vi "test-find-path-debug.vi"() -> ()   [LabVIEW 2019]
uses:
  <vilib>/Rock Robotics/WPI/ThirdParty/JAS_Junk/TrajLib/TypeDef/TRANSLATION2D.ctl
  <vilib>/Rock Robotics/WPI/ThirdParty/MJansen/PathPlanner/TypeDef/PathPlannerGoalEndState.ctl
  <vilib>/Rock Robotics/WPI/ThirdParty/JAS_Junk/TrajLib/TypeDef/ROTATION2D.ctl
  <vilib>/Rock Robotics/WPI/ThirdParty/MJansen/PathPlanner/TypeDef/PathPlannerPath.ctl
  <vilib>/Rock Robotics/WPI/ThirdParty/MJansen/PathPlanner/TypeDef/PathPlannerRotationTarget.ctl
  <vilib>/Rock Robotics/WPI/ThirdParty/MJansen/PathPlanner/TypeDef/PathPlannerConstraintsZone.ctl
  <vilib>/Rock Robotics/WPI/ThirdParty/MJansen/PathPlanner/TypeDef/PathPlannerPathConstraints.ctl
  <vilib>/Rock Robotics/WPI/ThirdParty/MJansen/PathPlanner/TypeDef/PathPlannerEventMarker.ctl
  <vilib>/Rock Robotics/WPI/ThirdParty/MJansen/PathPlanner/TypeDef/PathPlannerCommandUtil.ctl
  <vilib>/Rock Robotics/WPI/ThirdParty/MJansen/PathPlanner/ENum/PathPlanner_CommandUtilType_ENUM.ctl
  <vilib>/Rock Robotics/WPI/ThirdParty/MJansen/PathPlanner/TypeDef/PathPlannerPathPoint.ctl
  <vilib>/Rock Robotics/WPI/ThirdParty/MJansen/PathPlanner/TypeDef/PathPlannerWaypoint.ctl
  <vilib>/Rock Robotics/WPI/ThirdParty/MJansen/PathPlanner/TypeDef/PathPlannerPointTowardsZone.ctl
  <vilib>/Rock Robotics/WPI/ThirdParty/MJansen/PathPlanner/TypeDef/PathPlannerIdealStartingState.ctl
  <vilib>/Rock Robotics/WPI/ThirdParty/JAS_Junk/TrajLib/TypeDef/CHASSIS_SPEEDS.ctl
  <vilib>/Rock Robotics/WPI/ThirdParty/MJansen/PathPlanner/VI/PathPlanner_GridPosition_Get.vi
  <vilib>/Rock Robotics/WPI/ThirdParty/JAS_Junk/TrajLib/Translation2d_Create.vi
  <vilib>/Rock Robotics/WPI/ThirdParty/MJansen/PathPlanner/VI/PathPlanner_PathFinder_Globals.vi
  <vilib>/robotics/Navigation/shared/WorldMap/OccupancyGridWorldMap/NI_Robotics_OccupancyGridWorldMap.lvclass
  <vilib>/robotics/Navigation/shared/MapNode/AbstractDstarNode/NI_Robotics_AbstractDstarNode.lvclass
  <vilib>/Rock Robotics/WPI/ThirdParty/MJansen/PathPlanner/PathPlanner24.lvlib
  <vilib>/Rock Robotics/WPI/ThirdParty/JAS_Junk/TrajLib/Trajectory_Library.lvlib
panel:
  out "Loop Count 2":i32
  out "Extract Simplified Path Size":i32
  out "Do Reset Err Count":i64
  out "Do Minor Err Count":i64
  out "Do Major Err Count":i64
  out "Extract Path Size":i32
  out "Field":cluster{dbl[], dbl[]}[](graph)
  out "Error_No_Path":bool
  out "New Path Available":bool
  out "Loop Count":i32
  out "TerminateWorker":bool
  out "Do Work Count":i64
  out "Do Reset Count":i64
  out "Do Minor Count":i64
  out "Do Major Count":i64
  out "PathPlannerPath":T1={"Reversed"=FALSE, "RotationTargets"=[], "ConstraintZones"=[], "EventMarkers"=[], "GlobalConstraints"={"MaxVelocityMps;"=0.0, "MaxAccelerationMpsSq;"=0.0, "MaxAngularVelRadPsEc;"=0.0, "MaxAngularAccRadPSecSq"=0.0, "Exists"=FALSE, "Unlimited"=FALSE, "NominalVoltageVolts"=1.0}, "GoalEndState"={"VelocityMPS"=0.0, "Rotation"={"VALUE"=0.0, "COS"=1.0, "SIN"=0.0}}, "AllPoints"=[], "Name"="", "Waypoints"=[], "PointTowardsZones"=[], "IdealStartingState"={"VelocityMPS"=0.0, "Rotation"={"VALUE"=0.0, "COS"=1.0, "SIN"=0.0}}, "IsChoreoPath"=FALSE, "PreventFlipping"=FALSE} {"IdealStartingState"."Rotation"."SIN" format="%13.4f"; "IdealStartingState"."Rotation"."COS" format="%13.4f"; "IdealStartingState"."Rotation"."VALUE" format="%13.4f"; "PointTowardsZones"."TargetPosition"."Y" format="%14.3f"; "PointTowardsZones"."TargetPosition"."X" format="%14.3f"; "PointTowardsZones"."RotationOffset"."SIN" format="%13.4f"; "PointTowardsZones"."RotationOffset"."COS" format="%13.4f"; "PointTowardsZones"."RotationOffset"."VALUE" format="%13.4f"; "Waypoints"."nextControl"."Y" format="%14.3f"; "Waypoints"."nextControl"."X" format="%14.3f"; "Waypoints"."anchor"."Y" format="%14.3f"; "Waypoints"."anchor"."X" format="%14.3f"; "Waypoints"."prevControl"."Y" format="%14.3f"; "Waypoints"."prevControl"."X" format="%14.3f"; "AllPoints"."RotationTarget"."rotation"."SIN" format="%13.4f"; "AllPoints"."RotationTarget"."rotation"."COS" format="%13.4f"; "AllPoints"."RotationTarget"."rotation"."VALUE" format="%13.4f"; "AllPoints"."Position"."Y" format="%14.3f"; "AllPoints"."Position"."X" format="%14.3f"; "GoalEndState"."Rotation"."SIN" format="%13.4f"; "GoalEndState"."Rotation"."COS" format="%13.4f"; "GoalEndState"."Rotation"."VALUE" format="%13.4f"; "RotationTargets"."rotation"."SIN" format="%13.4f"; "RotationTargets"."rotation"."COS" format="%13.4f"; "RotationTargets"."rotation"."VALUE" format="%13.4f"}
  in  "GoalEndState":T9={"VelocityMPS"=0.0, "Rotation"={"VALUE"=0.0, "COS"=1.0, "SIN"=0.0}} {"Rotation"."SIN" format="%13.4f"; "Rotation"."COS" format="%13.4f"; "Rotation"."VALUE" format="%13.4f"}
  in  "Goal Position":T11={"X"=14.0, "Y"=7.0} {"Y" step=0.25 format="%14.3f"; "X" step=0.25 format="%14.3f"}
  in  "StartPosition":T11={"X"=1.5, "Y"=1.5} {"Y" step=0.25 format="%14.3f"; "X" step=0.25 format="%14.3f"}
  out "NewPathAvailLastCheck":i32
  out "NewPathAvailCount":i32
  out "BackGroundInitialized":bool
  out "Main Program Name":string
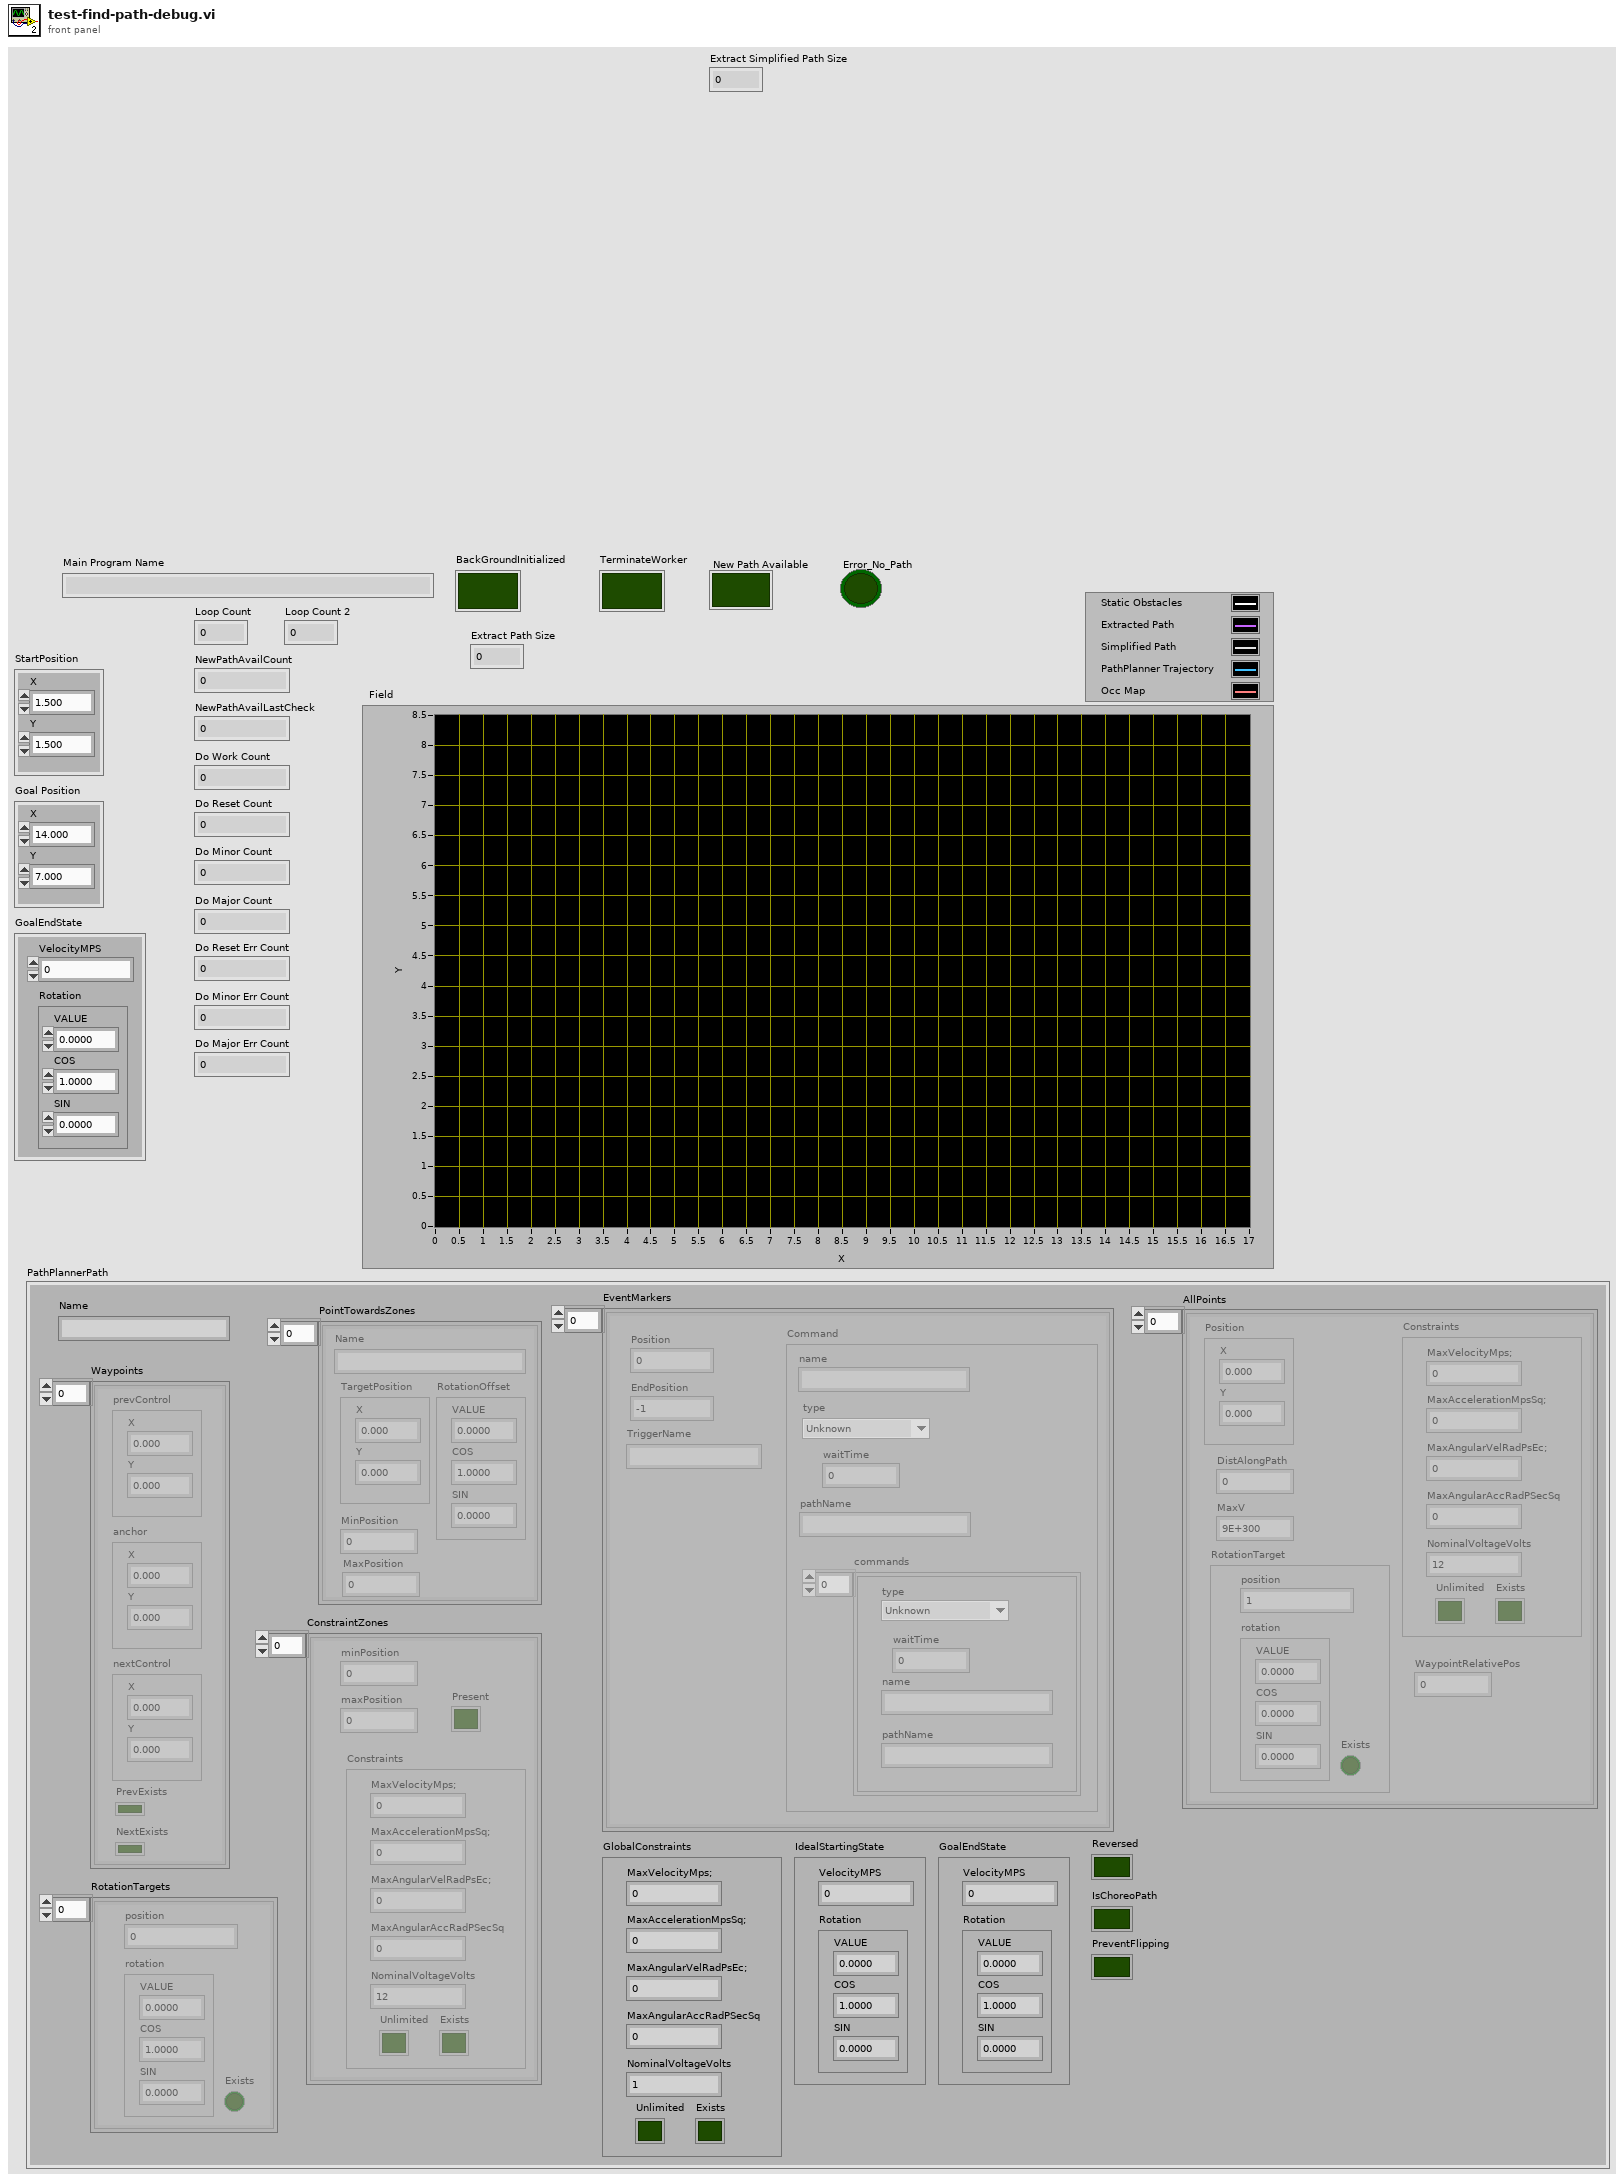
[diagram p1: front panel]
types:
  T1 = typedef "PathPlanner24.lvlib/PathPlannerPath.ctl" = cluster{"Reversed":bool, "RotationTargets":T2[], "ConstraintZones":T4[], "EventMarkers":T6[], "GlobalConstraints":T5, "GoalEndState":T9, "AllPoints":T10[], "Name":string, "Waypoints":T12[], "PointTowardsZones":T13[], "IdealStartingState":T14, "IsChoreoPath":bool, "PreventFlipping":bool}
  T2 = typedef "PathPlanner24.lvlib/PathPlannerRotationTarget.ctl" = cluster{"position":dbl, "rotation":T3, "Exists":bool}
  T3 = typedef "Trajectory_Library.lvlib/ROTATION2D.ctl" = cluster{"VALUE":dbl, "COS":dbl, "SIN":dbl}
  T4 = typedef "PathPlanner24.lvlib/PathPlannerConstraintsZone.ctl" = cluster{"minPosition":dbl, "maxPosition":dbl, "Constraints":T5, "Present":bool}
  T5 = typedef "PathPlanner24.lvlib/PathPlannerPathConstraints.ctl" = cluster{"MaxVelocityMps;":dbl, "MaxAccelerationMpsSq;":dbl, "MaxAngularVelRadPsEc;":dbl, "MaxAngularAccRadPSecSq":dbl, "Exists":bool, "Unlimited":bool, "NominalVoltageVolts":dbl}
  T6 = typedef "PathPlanner24.lvlib/PathPlannerEventMarker.ctl" = cluster{"Position":dbl, "Command":T7, "TriggerName":string, "EndPosition":dbl}
  T7 = typedef "PathPlanner24.lvlib/PathPlannerCommandUtil.ctl" = cluster{"waitTime":dbl, "name":string, "pathName":string, "commands":cluster{"type":T8, "waitTime":dbl, "name":string, "pathName":string}[], "type":T8}
  T8 = typedef "PathPlanner24.lvlib/PathPlanner_CommandUtilType_ENUM.ctl" = enum16{"Unknown", "Wait", "Named", "Path", "Sequential", "Parallel", "Race", "Deadline"}
  T9 = typedef "PathPlanner24.lvlib/PathPlannerGoalEndState.ctl" = cluster{"VelocityMPS":dbl, "Rotation":T3}
  T10 = typedef "PathPlanner24.lvlib/PathPlannerPathPoint.ctl" = cluster{"Position":T11, "DistAlongPath":dbl, "MaxV":dbl, "Constraints":T5, "RotationTarget":T2, "WaypointRelativePos":dbl}
  T11 = typedef "Trajectory_Library.lvlib/TRANSLATION2D.ctl" = cluster{"X":dbl, "Y":dbl}
  T12 = typedef "PathPlanner24.lvlib/PathPlannerWaypoint.ctl" = cluster{"prevControl":T11, "anchor":T11, "nextControl":T11, "PrevExists":bool, "NextExists":bool}
  T13 = typedef "PathPlanner24.lvlib/PathPlannerPointTowardsZone.ctl" = cluster{"RotationOffset":T3, "Name":string, "TargetPosition":T11, "MinPosition":dbl, "MaxPosition":dbl}
  T14 = typedef "PathPlanner24.lvlib/PathPlannerIdealStartingState.ctl" = cluster{"VelocityMPS":dbl, "Rotation":T3}
  T15 = cluster{"DoResetErrCount":i64, "DoResetCount":i64, "DoMinorErrCount":i64, "DoMinorCount":i64, "DoMajorErrCount":i64, "DoMajorCount":i64, "DoWorkLoopCount":i64, "BackGroundInitialized":bool, "TerminateWorker":bool}
  T16 = typedef "Trajectory_Library.lvlib/CHASSIS_SPEEDS.ctl" = cluster{"vX":dbl, "vY":dbl, "vOmega":dbl}
  T17 = typedef "PathPlanner24.lvlib/PathPlannerFinderGridPosition.ctl" = cluster{"X":i32, "Y":i32}
  T18 = cluster{"ExtractedPath":T17[], "ExtractedPathSimplified":T17[], "ExtractedFieldPosPath":T11[], "CurrentPath":T11[], "Obstacles":set{T17}, "StaticOccupancyGrid":refnum<data-value>, "path references":refnum<data-value>[], "Main Program Name":string}
  T19 = typedef "PathPlanner24.lvlib/PathPlannerTrajectory.ctl" = cluster{"States":T20[]}
  T20 = typedef "PathPlanner24.lvlib/PathPlannerTrajectoryState.ctl" = cluster{"TimeSeconds":dbl, "VelocityMPS":dbl, "AccerationMpsSq":dbl, "HeadingAngularVelRadPerSec":dbl, "PositionMeters":T11, "Heading":T3, "TargetHolonomicRotation":T3, "CurvatureRadPerMeter":dbl, "PathPlannerConstraints":T5, "DeltaPos":dbl}
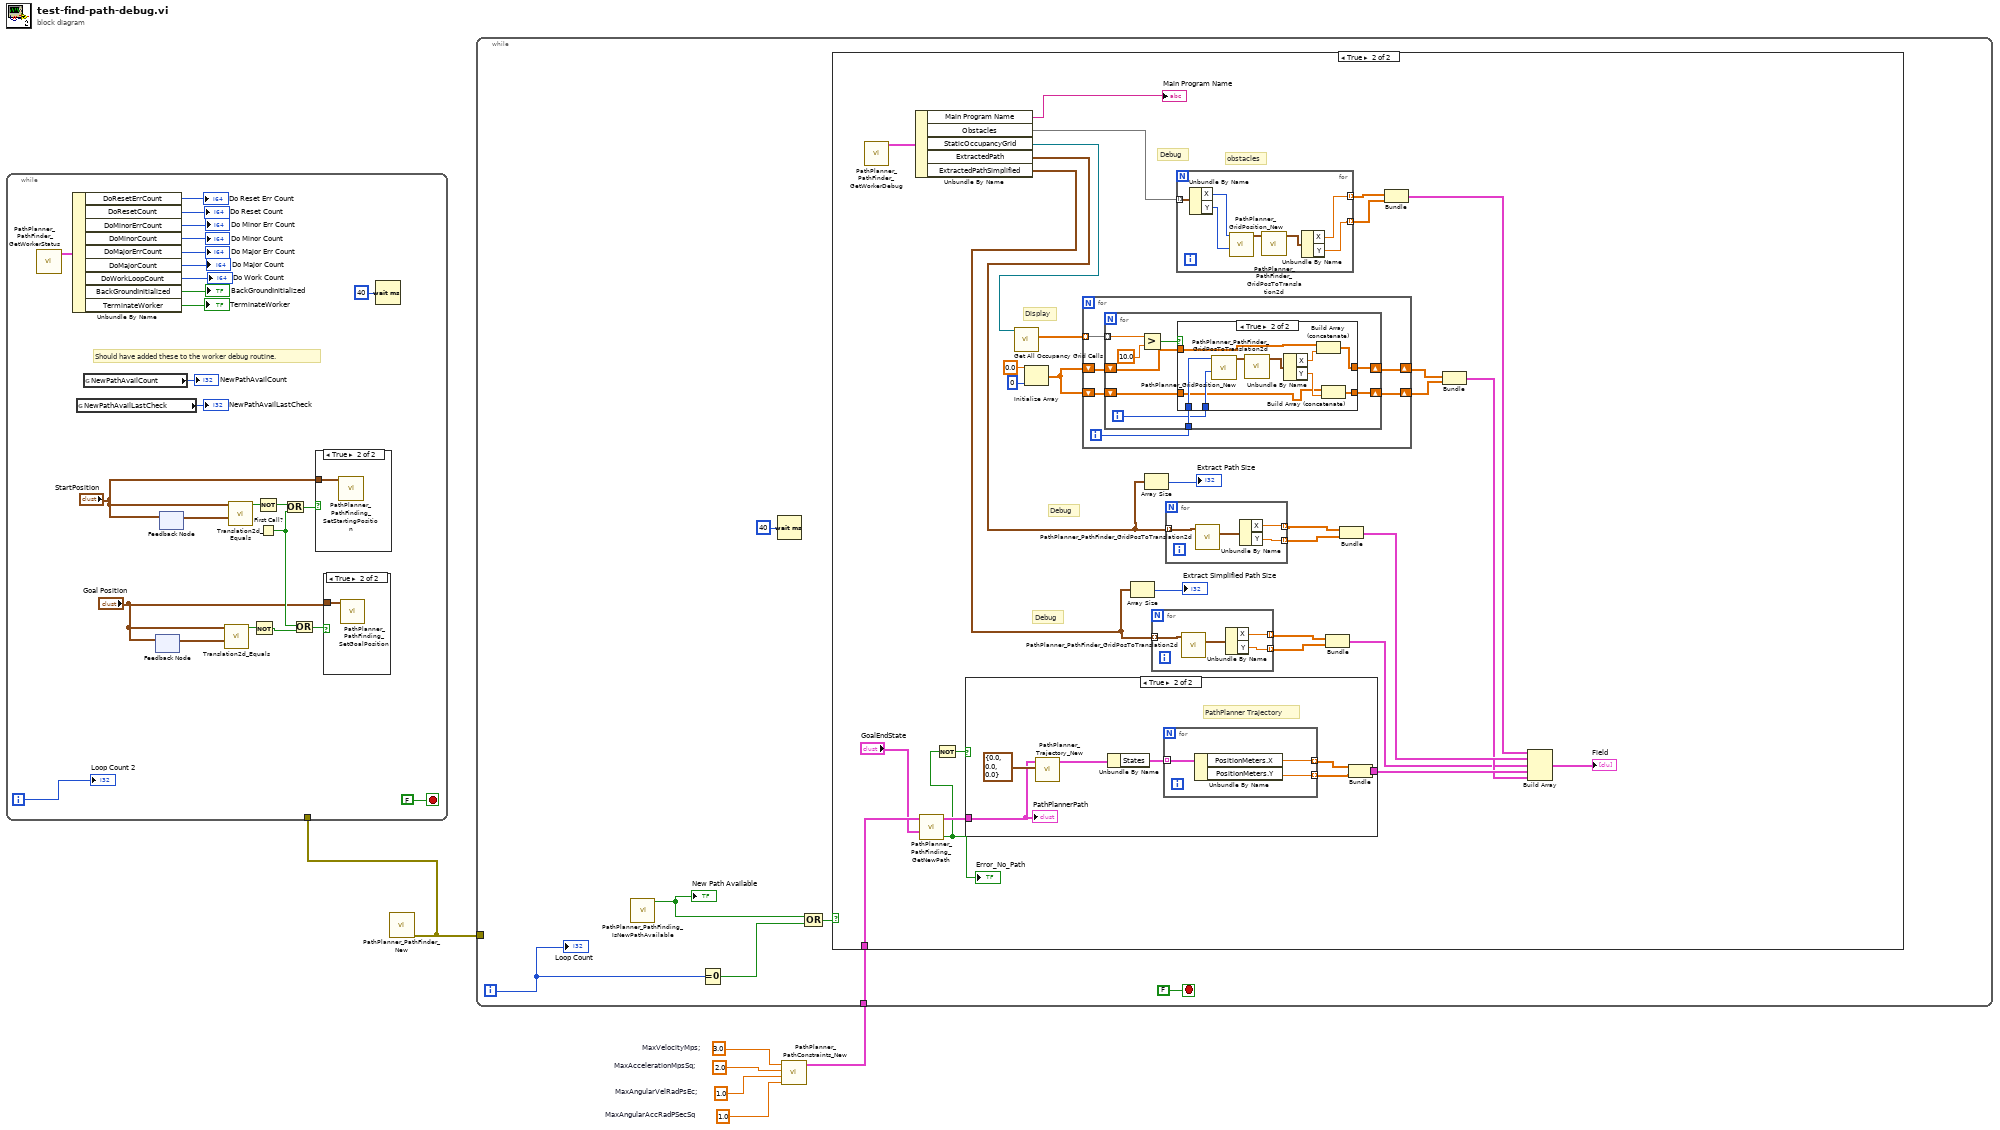
[diagram p0: block diagram]
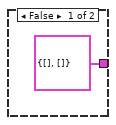
[diagram p5: hidden frame]
diagram:
  w2 = 3.0  # MaxVelocityMps;
  w3 = 2.0  # MaxAccelerationMpsSq;
  w4 = 1.0  # MaxAngularVelRadPsEc;
  w5 = 1.0  # MaxAngularAccRadPSecSq
  n1 = call <vilib>:"PathPlanner_PathFinder_New.vi"() -> ("error out"=w1:errorcluster)  [unwired: 11 in]
  n2 = while {
    tunnel: w1 -> [_]
    i -> [w18]
    stop <- FALSE stop-if-true
    # "Should have added these to the worker debug routine."
    n3 = call <vilib>:"PathPlanner_PathFinder_GetWorkerStatus.vi"() -> ("PathFindingWorkerStatus"=w23:T15)  [unwired: 11 in]
    n4 = Unbundle By Name(w23) -> ("DoResetErrCount"=→"Do Reset Err Count":i64, "DoResetCount"=→"Do Reset Count":i64, "DoMinorErrCount"=→"Do Minor Err Count":i64, "DoMinorCount"=→"Do Minor Count":i64, "DoMajorErrCount"=→"Do Major Err Count":i64, "DoMajorCount"=→"Do Major Count":i64, "DoWorkLoopCount"=→"Do Work Count":i64, "BackGroundInitialized"=→"BackGroundInitialized":bool, "TerminateWorker"=→"TerminateWorker":bool)
    n5 = global read "PathPlanner_PathFinder_Globals.vi" "NewPathAvailLastCheck"() -> (→"NewPathAvailLastCheck":i32)
    n6 = global read "PathPlanner_PathFinder_Globals.vi" "NewPathAvailCount"() -> (→"NewPathAvailCount":i32)
    n7 = feedback #1() -> (w9:T11)  [unwired: 1 in]
    n8 = feedback-in #1("Goal Position") -> ()
    n9 = feedback #2() -> (w7:T11)  [unwired: 1 in]
    n10 = feedback-in #2("StartPosition") -> ()
    n11 = call <vilib>:"Translation2d_Equals.vi"("other Translation"=w9, "In Translation"="Goal Position") -> ("Equals"=w10:bool)  [unwired: 9 in]
    n12 = call <vilib>:"Translation2d_Equals.vi"("other Translation"=w7, "In Translation"="StartPosition") -> ("Equals"=w8:bool)  [unwired: 9 in]
    n13 = Not(x=w10) -> (.not. x?=w15:bool)
    n14 = Not(x=w8) -> (.not. x?=w17:bool)
    n15 = First Call?() -> (First Call?: T/F=w16:bool)
    n16 = Or(x=w17, y=w16) -> (x .or. y?=w13:bool)
    n17 = Or(x=w16, y=w15) -> (x .or. y?=w14:bool)
    n18 = case shown="True" w13 {
      tunnel: "StartPosition" -> [_ w34]
      frame False {
      }
      frame True {
        n19 = call <vilib>:"PathPlanner_PathFinding_SetStartingPosition.vi"("StartPosition"=w34) -> ()  [unwired: 10 in, 1 out]
      }
    }
    n20 = case shown="True" w14 {
      tunnel: "Goal Position" -> [_ w33]
      frame False {
      }
      frame True {
        n21 = call <vilib>:"PathPlanner_PathFinding_SetGoalPosition.vi"("GoalPosition"=w33) -> ()  [unwired: 10 in, 1 out]
      }
    }
    n22 = Wait (ms)(milliseconds to wait=u32 40) -> ()  [unwired: 1 out]
    "Loop Count 2" <- w18
  }
  n23 = call <vilib>:"PathPlanner_PathConstraints_New.vi"("MaxAngularAccRadPSecSq"=w5, "MaxAngularVelRadPsEc;"=w4, "MaxAccelerationMpsSq;"=w3, "MaxVelocityMps;"=w2) -> ("PathPlannerConstraints"=w6:T5)  [unwired: 7 in]
  n24 = while {
    tunnel: w6 -> [w38]
    tunnel: w1 -> [_]
    i -> [w40]
    stop <- FALSE stop-if-true
    n25 = call <vilib>:"PathPlanner_PathFinding_IsNewPathAvailable.vi"() -> ("New Path Available"=w35:bool)  [unwired: 10 in, 1 out]
    "New Path Available" <- w35
    n26 = Equal To 0?(x=w40) -> (x = 0?=w37:bool)
    n27 = Wait (ms)(milliseconds to wait=u32 40) -> ()  [unwired: 1 out]
    n28 = Compound Arithmetic op=OR(w35, w37) -> (w39:bool)
    n29 = case shown="True" w39 {
      tunnel: w38 -> [_ w67]
      frame False {
      }
      frame True {
        # "Debug"
        # "Display"
        # "Debug"
        # "Debug"
        # "obstacles"
        n30 = call <vilib>:"PathPlanner_PathFinder_GetWorkerDebug.vi"() -> ("PathFinderWorkerDebug"=w49:T18)  [unwired: 11 in]
        n31 = Unbundle By Name(w49) -> ("Main Program Name"=→"Main Program Name":string, "Obstacles"=w47:set{T17}, "StaticOccupancyGrid"=w46:refnum<data-value>, "ExtractedPath"=w45:T17[], "ExtractedPathSimplified"=w44:T17[])
        n32 = call <vilib>:"PathPlanner_PathFinding_GetNewPath.vi"("GoalEndState"="GoalEndState", "PathPlannerPathConstraints"=w67) -> ("Error_No_Path"=w42:bool, "PathPlannerPath"=w65:T1)  [unwired: 8 in]
        "Error_No_Path" <- w42
        n33 = Not(x=w42) -> (.not. x?=w43:bool)
        n34 = case shown="True" w43 {
          tunnel: w65 -> [_ w78]
          tunnel: [cluster{dbl[], dbl[]} {[], []} w74] -> w62
          frame False {
          }
          frame True {
            # "PathPlanner Trajectory"
            n35 = call <vilib>:"PathPlanner_Trajectory_New.vi"("StartingSpeeds"=T16 {"vX"=0.0, "vY"=0.0, "vOmega"=0.0}, "Path"=w78) -> ("PathPlannerTrajectory"=w79:T19)  [unwired: 8 in, 1 out]
            n36 = Unbundle By Name(w79) -> ("States"=w77:T20[])
            n37 = for {
              tunnel: [w82] -> w76 mode=indexing
              tunnel: [w83] -> w75 mode=indexing
              tunnel: w77 -> [w81] mode=indexing
              n38 = Unbundle By Name(w81) -> ("PositionMeters.X"=w82:dbl, "PositionMeters.Y"=w83:dbl)
            }
            n39 = Bundle(w76, w75) -> (w74:cluster{dbl[], dbl[]})  [unwired: 1 in]
            "PathPlannerPath" <- w78
          }
        }
        n40 = call <vilib>:"Get All Occupancy Grid Cells.vi"("map reference in"=w46) -> ("occupancy grid"=w53:dbl[][])  [unwired: 8 in, 2 out]
        n41 = Initialize Array(0.0 ("element"), 0 ("dimension size")) -> (w50:dbl[])
        n42 = for {
          tunnel: w53 -> [w93] mode=indexing
          shift-right: [w89] -> w60
          shift-left: w50 -> [w92]
          shift-right: [w88] -> w59
          shift-left: w50 -> [w91]
          i -> [w90]
          n43 = for {
            tunnel: w93 -> [w102] mode=indexing
            shift-right: [w96] -> w89
            shift-left: w92 -> [w97]
            shift-right: [w94] -> w88
            shift-left: w91 -> [w95]
            tunnel: w90 -> [w99]
            i -> [w98]
            n44 = Greater?(x=w102, y=10.0) -> (0:w100:bool)
            n45 = case shown="True" w100 {
              tunnel: w99 -> [_ w113]
              tunnel: w98 -> [_ w109]
              tunnel: w97 -> [w104 w108]
              tunnel: [w104 w107] -> w96
              tunnel: w95 -> [w103 w106]
              tunnel: [w103 w105] -> w94
              frame False {
              }
              frame True {
                n46 = call <vilib>:"PathPlanner_GridPosition_New.vi"("Int Y"=w109, "Int X"=w113) -> ("GridPosition"=w114:T17)  [unwired: 9 in]
                n47 = call <vilib>:"PathPlanner_PathFinder_GridPosToTranslation2d.vi"("GridPosition"=w114) -> ("RealGridPos"=w112:T11)  [unwired: 10 in]
                n48 = Unbundle By Name(w112) -> ("X"=w111:dbl, "Y"=w110:dbl)
                n49 = Build Array (concatenate)(w108, w111) -> (w107:dbl[])
                n50 = Build Array (concatenate)(w106, w110) -> (w105:dbl[])
              }
            }
          }
        }
        n51 = Array Size(array=w44) -> (size(s)=→"Extract Simplified Path Size":i32)
        n52 = Array Size(array=w45) -> (size(s)=→"Extract Path Size":i32)
        n53 = for {
          tunnel: [w85] -> w57 mode=indexing
          tunnel: [w87] -> w56 mode=indexing
          tunnel: w44 -> [w84] mode=indexing
          n54 = call <vilib>:"PathPlanner_PathFinder_GridPosToTranslation2d.vi"("GridPosition"=w84) -> ("RealGridPos"=w86:T11)  [unwired: 10 in]
          n55 = Unbundle By Name(w86) -> ("X"=w85:dbl, "Y"=w87:dbl)
        }
        n56 = for {
          tunnel: [w116] -> w64 mode=indexing
          tunnel: [w118] -> w63 mode=indexing
          tunnel: w45 -> [w115] mode=indexing
          n57 = call <vilib>:"PathPlanner_PathFinder_GridPosToTranslation2d.vi"("GridPosition"=w115) -> ("RealGridPos"=w117:T11)  [unwired: 10 in]
          n58 = Unbundle By Name(w117) -> ("X"=w116:dbl, "Y"=w118:dbl)
        }
        n59 = for {
          tunnel: w47 -> [w125] mode=indexing
          tunnel: [w120] -> w71 mode=indexing
          tunnel: [w119] -> w72 mode=indexing
          n60 = Unbundle By Name(w125) -> ("X"=w122:i32, "Y"=w121:i32)
          n61 = call <vilib>:"PathPlanner_GridPosition_New.vi"("Int Y"=w121, "Int X"=w122) -> ("GridPosition"=w124:T17)  [unwired: 9 in]
          n62 = call <vilib>:"PathPlanner_PathFinder_GridPosToTranslation2d.vi"("GridPosition"=w124) -> ("RealGridPos"=w123:T11)  [unwired: 10 in]
          n63 = Unbundle By Name(w123) -> ("X"=w120:dbl, "Y"=w119:dbl)
        }
        n64 = Bundle(w57, w56) -> (w54:cluster{dbl[], dbl[]})  [unwired: 1 in]
        n65 = Bundle(w64, w63) -> (w68:cluster{dbl[], dbl[]})  [unwired: 1 in]
        n66 = Bundle(w71, w72) -> (w69:cluster{dbl[], dbl[]})  [unwired: 1 in]
        n67 = Bundle(w60, w59) -> (w61:cluster{dbl[], dbl[]})  [unwired: 1 in]
        n68 = Build Array(w69, w68, w54, w62, w61) -> (→"Field":cluster{dbl[], dbl[]}[])
      }
    }
    "Loop Count" <- w40
  }
